vi "Configure Compass Orientation.vi"(8 "error in (no error)":errorcluster, 10 "Mount Orientation ( Flat )":dbl(ring)=1.0 items=["Standard-flat"=1.0, "Front"=2.0, "Port"=3.0, "Roof"=4.0, "Back"=5.0, "StarBoard"=6.0], 11 "VISA resource name":refnum<visa-resource-name>) -> (0 "error out":errorcluster, 3 "VISA resource out":refnum<visa-resource-name>)   [LabVIEW 2011, in "Ocean Server OS4000.lvlib"]
doc: "Configures the intrument to be set at six mounting orientations."
uses:
  Ocean Server OS4000.lvlib
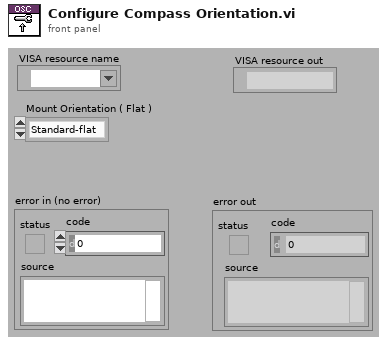
[diagram p1: front panel]
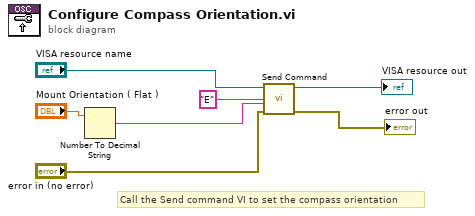
[diagram p0: block diagram]
diagram:
  # "Call the Send command VI to set the compass orientation"
  n1 = Number To Decimal String(number="Mount Orientation ( Flat )") -> (decimal integer string=w4:string)  [unwired: 1 in]
  n2 = call "Send Command.vi"("error in (no error)"="error in (no error)", "Value"=w4, "Message"="E", "VISA resource name"="VISA resource name") -> ("error out"=→"error out":errorcluster, "VISA resource out"=→"VISA resource out":refnum<visa-resource-name>)  [unwired: 6 in]
